vi "点位计算软件.vi"() -> ()   [LabVIEW 2020]
panel:
  in  "计算":bool
  out "error out":errorcluster
  in  "保存路径":path=path "D:/上下限/输入输出.ini" caption="配置文件的路径"
  in  "保存":bool
  in  "退出":bool
  in  "Tab Control":T1(tab)
  in  "Y 13":dbl
  in  "X 13":dbl
  in  "Y 12":dbl
  in  "X 12":dbl
  in  "Y 11":dbl
  in  "X 11":dbl
  in  "Y 10":dbl
  in  "X 10":dbl
  in  "Y 9":dbl
  in  "X 9":dbl
  in  "Y 8":dbl
  in  "X 8":dbl
  in  "Y 7":dbl
  in  "X 7":dbl
  in  "Y 6":dbl
  in  "X 6":dbl
  in  "Y 4":dbl
  in  "X 4":dbl
  in  "Y 5":dbl
  in  "X 5":dbl
  in  "Y 3":dbl
  in  "X 3":dbl
  in  "X 2":dbl
  in  "Y 2":dbl
  in  "Y 1":dbl
  in  "X 1":dbl
  in  "Y0":dbl
  in  "X 0":dbl
  out "?":bool
  out "?":bool
  out "?":bool
  out "?":bool
  out "?":bool
  out "?":bool
  out "?":bool
  out "?":bool
  out "?":bool
  out "?":bool
  out "?":bool
  out "?":bool
  out "?":bool
  out "?":bool
  in  "右侧边缘X坐标":dbl=2000.0 format="%#.3f"
  in  "左侧边缘X坐标":dbl=1000.0
  in  "上侧边缘Y坐标":dbl=1000.0
  in  "下侧边缘Y坐标":dbl=2000.0
  in  "产品宽度":dbl=23.67 format="%#_13g"
  in  "产品长度":dbl=13.3 format="%#_13g"
  in  "左侧边缘X坐标":dbl=1000.0
  in  "右侧边缘X坐标":dbl=2000.0 format="%#.3f"
  in  "上侧边缘Y坐标":dbl=1000.0
  in  "下侧边缘Y坐标":dbl=2000.0
  in  "X 8":dbl
  in  "Y 8":dbl
  in  "X 7":dbl
  in  "Y 7":dbl
  in  "X 6":dbl
  in  "Y 6":dbl
  in  "X 5":dbl
  in  "Y 5":dbl
  in  "X 4":dbl
  in  "Y 4":dbl
  in  "X 3":dbl
  in  "Y 3":dbl
  in  "Y 2":dbl
  in  "X 2":dbl
  in  "X 1":dbl
  in  "Y 1":dbl
  in  "X 0":dbl
  in  "Y 0":dbl
  out "?":bool
  out "?":bool
  out "?":bool
  out "?":bool
  out "?":bool
  out "?":bool
  out "?":bool
  out "?":bool
  out "?":bool
  out "?":bool
  out "?":bool
  out "?":bool
  out "?":bool
  out "?":bool
  out "?":bool
  out "?":bool
  out "?":bool
  out "?":bool
  out "?":bool
  out "?":bool
  out "?":bool
  out "?":bool
  out "?":bool
  out "X 0":dbl format="%#.3f"
  out "Y 0":dbl format="%#.3f"
  out "X 1":dbl format="%#.3f"
  out "Y 1":dbl format="%#.3f"
  out "Y 2":dbl format="%#.3f"
  out "X 2":dbl format="%#.3f"
  out "X 3":dbl format="%#.3f"
  out "Y 3":dbl format="%#.3f"
  out "X 5":dbl format="%#.3f"
  out "Y 5":dbl format="%#.3f"
  out "X 4":dbl format="%#.3f"
  out "Y 4":dbl format="%#.3f"
  out "X 6":dbl format="%#.3f"
  out "Y 6":dbl format="%#.3f"
  out "X 7":dbl format="%#.3f"
  out "Y 7":dbl format="%#.3f"
  out "X 8":dbl format="%#.3f"
  out "Y 8":dbl format="%#.3f"
  out "X 9":dbl format="%#.3f"
  out "Y 9":dbl format="%#.3f"
  out "X 10":dbl format="%#.3f"
  out "Y 10":dbl format="%#.3f"
  out "X 11":dbl format="%#.3f"
  out "Y 11":dbl format="%#.3f"
  out "X 12":dbl format="%#.3f"
  out "Y 12":dbl format="%#.3f"
  out "X 13":dbl format="%#.3f"
  out "Y 13":dbl format="%#.3f"
  out "?":bool
  out "?":bool
  out "?":bool
  out "?":bool
  out "?":bool
  out "?":bool
  out "?":bool
  out "?":bool
  out "?":bool
  out "Y 0":dbl format="%#.3f"
  out "X 0":dbl format="%#.3f"
  out "Y 1":dbl format="%#.3f"
  out "X 1":dbl format="%#.3f"
  out "X 2":dbl format="%#.3f"
  out "Y 2":dbl format="%#.3f"
  out "Y 3":dbl format="%#.3f"
  out "X 3":dbl format="%#.3f"
  out "Y 4":dbl format="%#.3f"
  out "X 4":dbl format="%#.3f"
  out "Y 5":dbl format="%#.3f"
  out "X 5":dbl format="%#.3f"
  out "Y 6":dbl format="%#.3f"
  out "X 6":dbl format="%#.3f"
  out "Y 7":dbl format="%#.3f"
  out "X 7":dbl format="%#.3f"
  out "Y 8":dbl format="%#.3f"
  out "X 8":dbl format="%#.3f"
  out "Y 13":dbl format="%#.3f"
  out "X 13":dbl format="%#.3f"
  out "Y 12":dbl format="%#.3f"
  out "X 12":dbl format="%#.3f"
  out "Y 11":dbl format="%#.3f"
  out "X 11":dbl format="%#.3f"
  out "Y 10":dbl format="%#.3f"
  out "X 10":dbl format="%#.3f"
  out "Y 9":dbl format="%#.3f"
  out "X 9":dbl format="%#.3f"
  out "Y 8":dbl format="%#.3f"
  out "X 8":dbl format="%#.3f"
  out "Y 7":dbl format="%#.3f"
  out "X 7":dbl format="%#.3f"
  out "Y 6":dbl format="%#.3f"
  out "X 6":dbl format="%#.3f"
  out "Y 4":dbl format="%#.3f"
  out "X 4":dbl format="%#.3f"
  out "Y 5":dbl format="%#.3f"
  out "X 5":dbl format="%#.3f"
  out "Y 3":dbl format="%#.3f"
  out "X 3":dbl format="%#.3f"
  out "X 2":dbl format="%#.3f"
  out "Y 2":dbl format="%#.3f"
  out "Y 1":dbl format="%#.3f"
  out "X 1":dbl format="%#.3f"
  out "Y 0":dbl format="%#.3f"
  out "X 0":dbl format="%#.3f"
  out "?":bool
  out "?":bool
  out "?":bool
  out "?":bool
  out "?":bool
  out "?":bool
  out "?":bool
  out "?":bool
  out "?":bool
  out "?":bool
  out "?":bool
  out "?":bool
  out "?":bool
  out "?":bool
  out "X 8":dbl format="%#.3f"
  out "Y 8":dbl format="%#.3f"
  out "X 7":dbl format="%#.3f"
  out "Y 7":dbl format="%#.3f"
  out "X 6":dbl format="%#.3f"
  out "Y 6":dbl format="%#.3f"
  out "X 5":dbl format="%#.3f"
  out "Y 5":dbl format="%#.3f"
  out "X 4":dbl format="%#.3f"
  out "Y 4":dbl format="%#.3f"
  out "X 3":dbl format="%#.3f"
  out "Y 3":dbl format="%#.3f"
  out "Y 2":dbl format="%#.3f"
  out "X 2":dbl format="%#.3f"
  out "X 1":dbl format="%#.3f"
  out "Y 1":dbl format="%#.3f"
  out "X 0":dbl format="%#.3f"
  out "Y 0":dbl format="%#.3f"
  out "?":bool
  out "?":bool
  out "?":bool
  out "?":bool
  out "?":bool
  out "?":bool
  out "?":bool
  out "?":bool
  out "?":bool
  # "产品1"
  # "产品2"
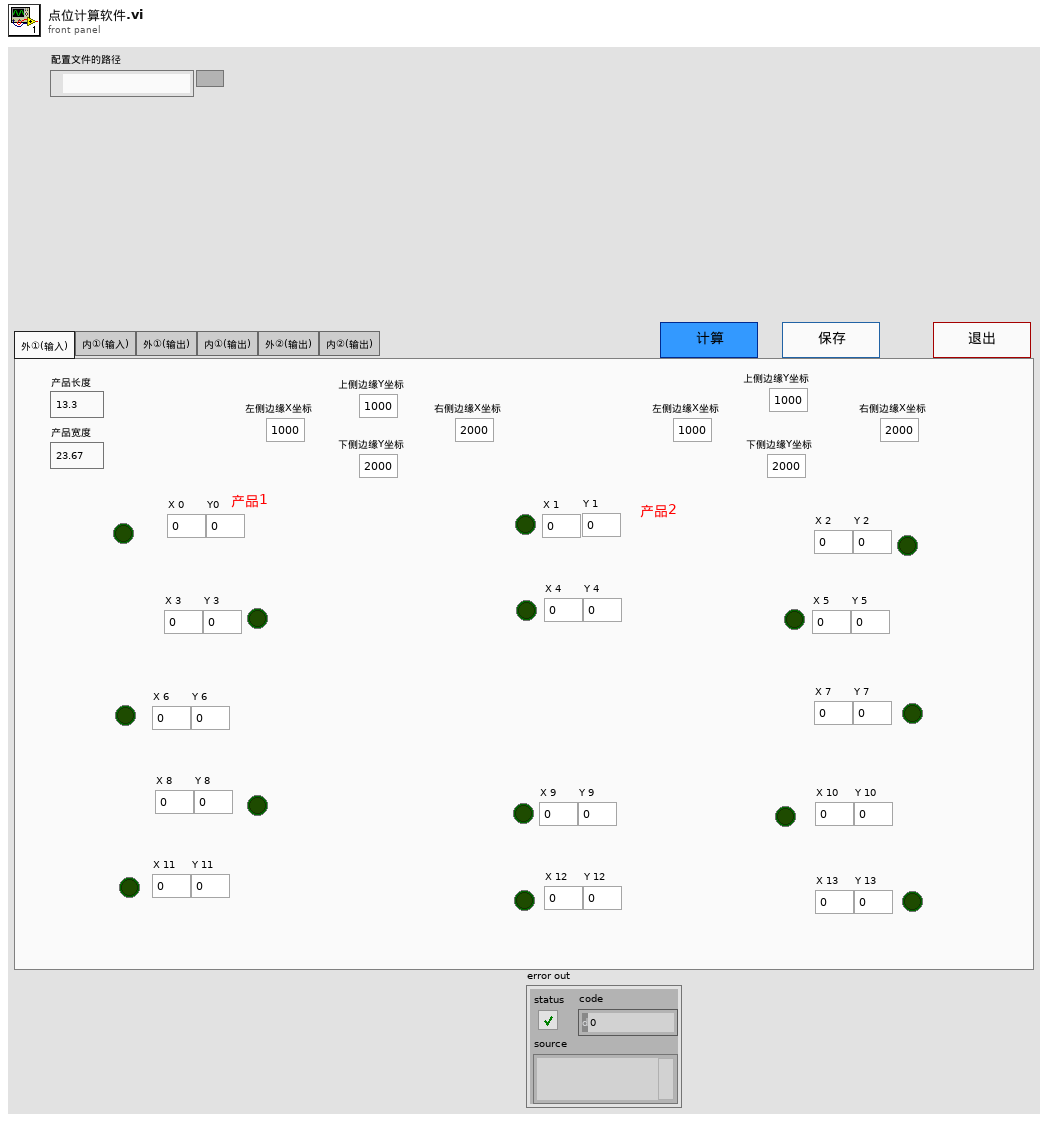
[diagram p1: front panel]
types:
  T1 = enum32{"外①(输入)", "内①(输入)", "外①(输出)", "内①(输出)", "外②(输出)", "内②(输出)"}
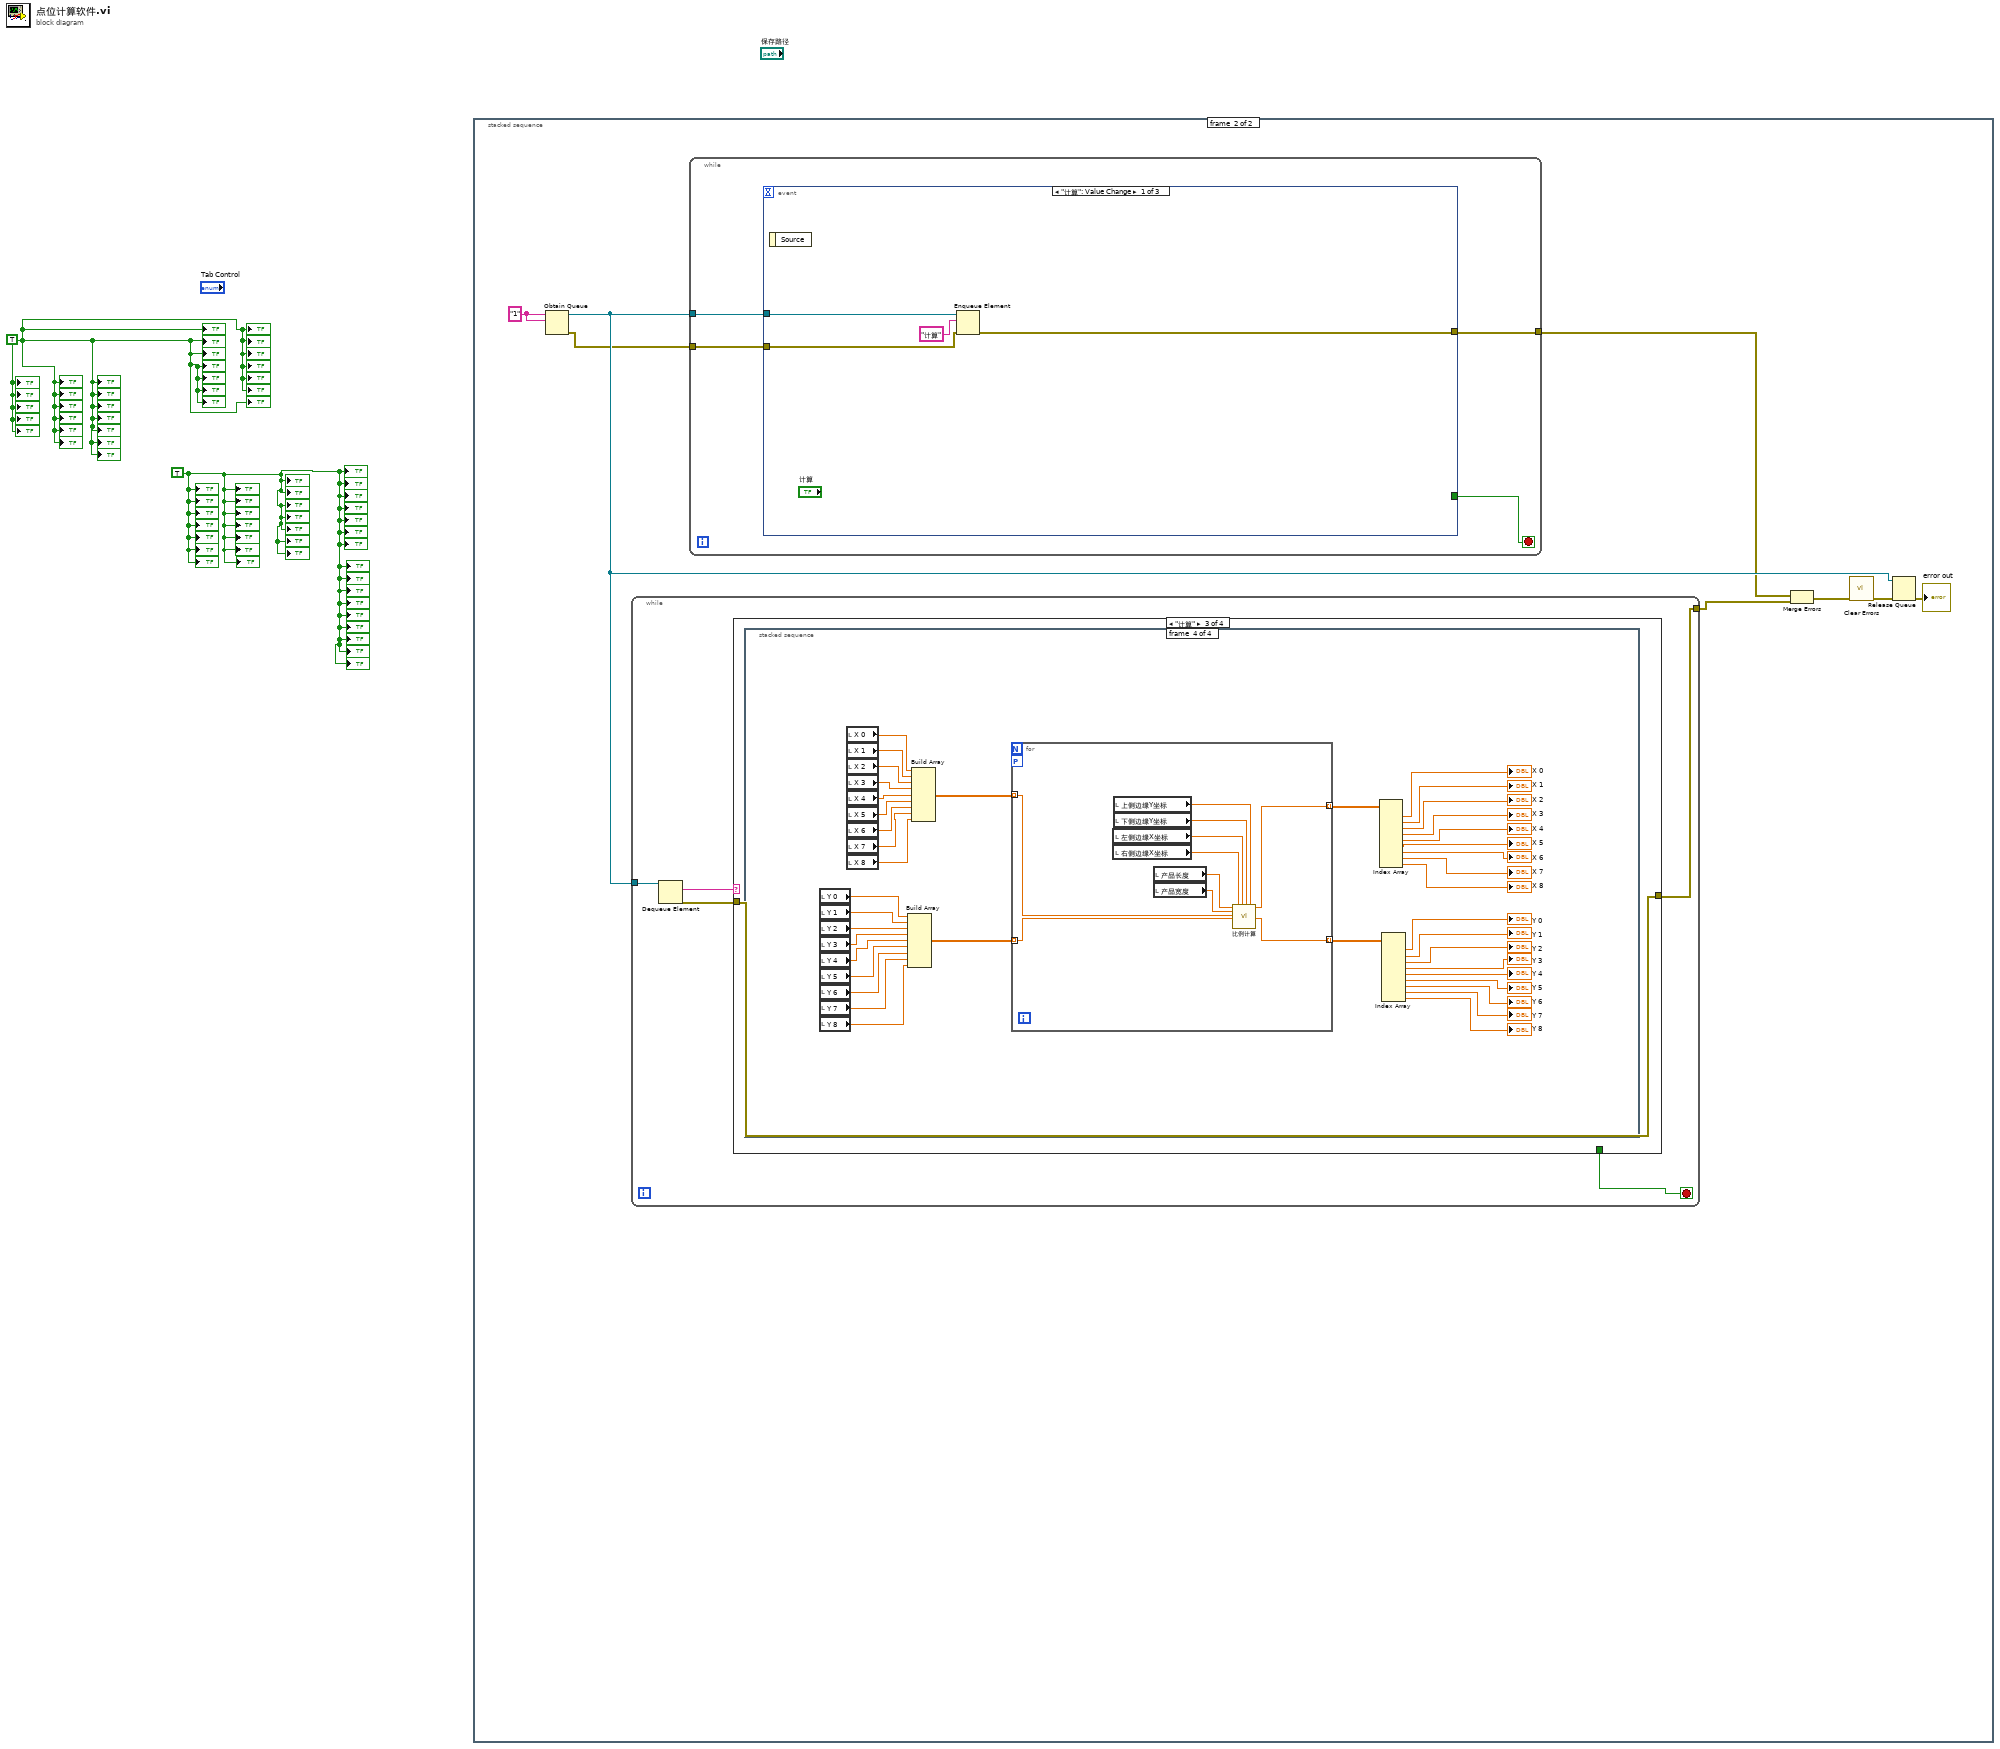
[diagram p0: block diagram]
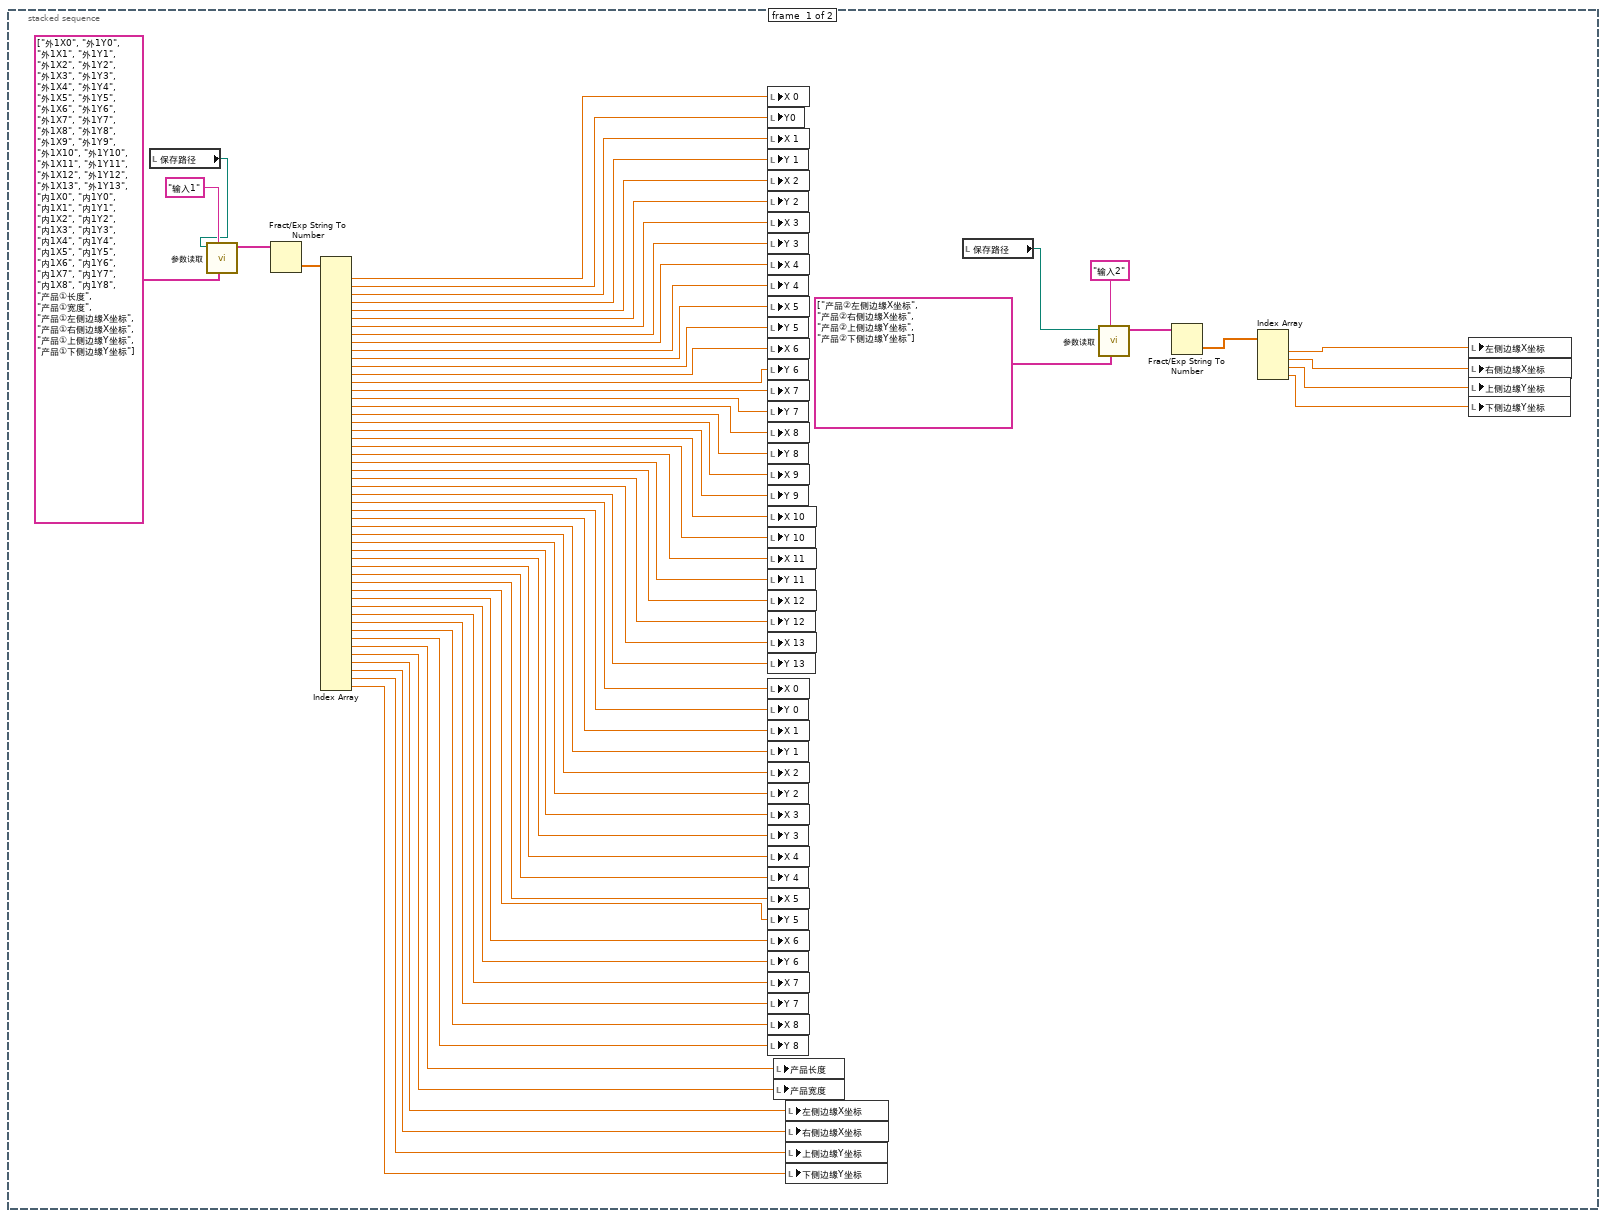
[diagram p2: hidden frame]
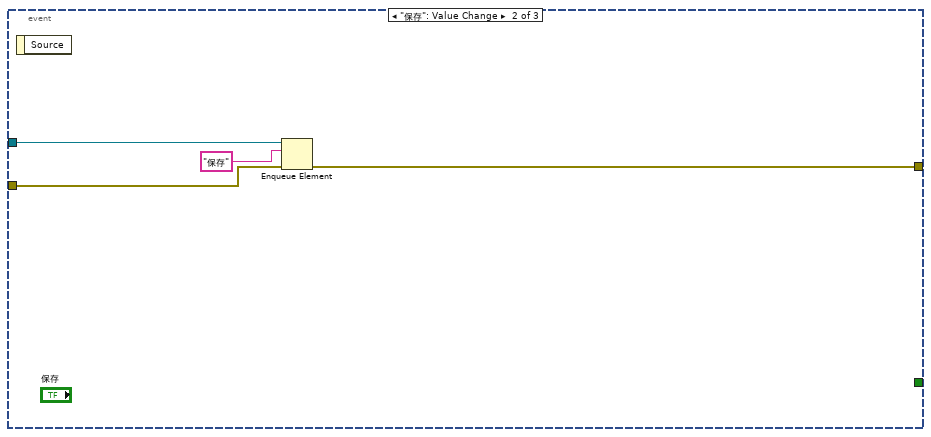
[diagram p3: hidden frame]
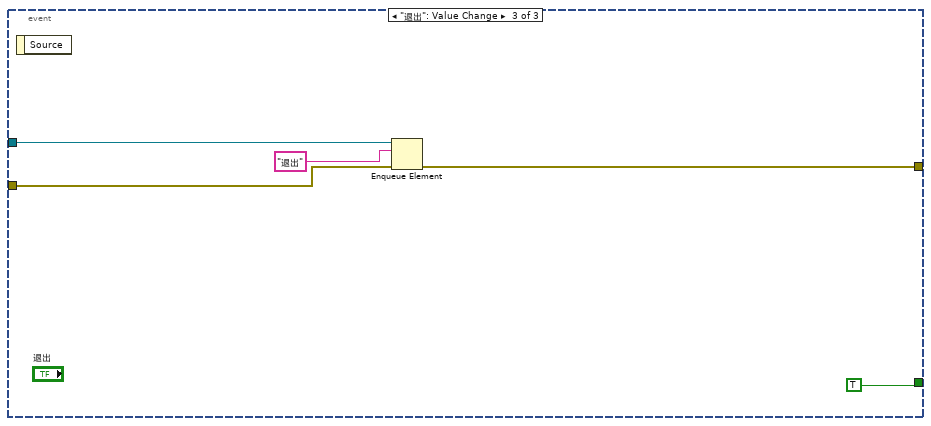
[diagram p4: hidden frame]
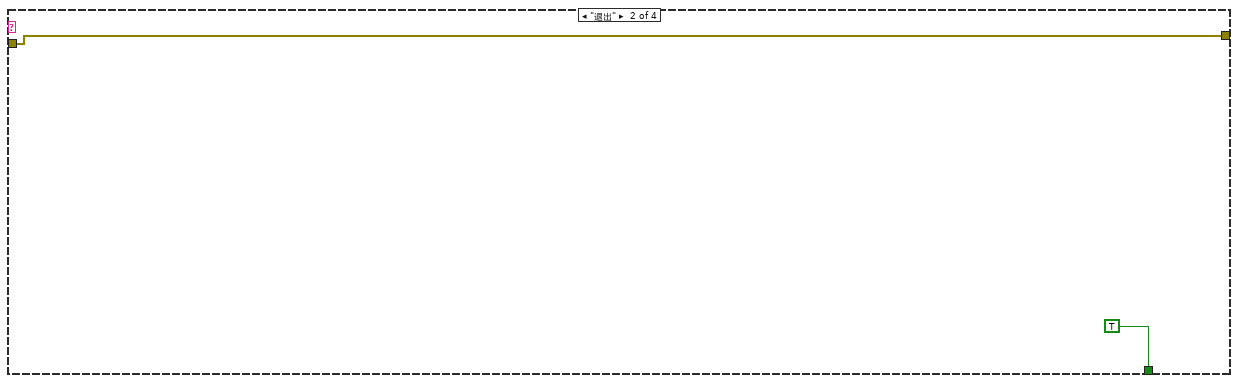
[diagram p6: hidden frame]
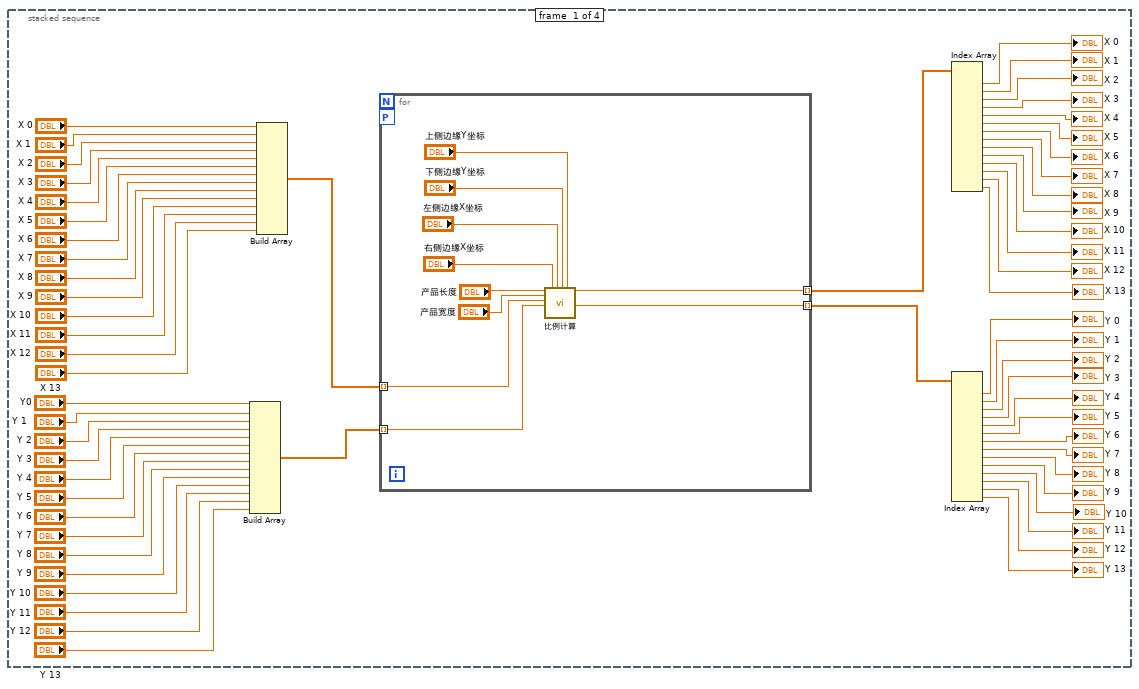
[diagram p7: hidden frame]
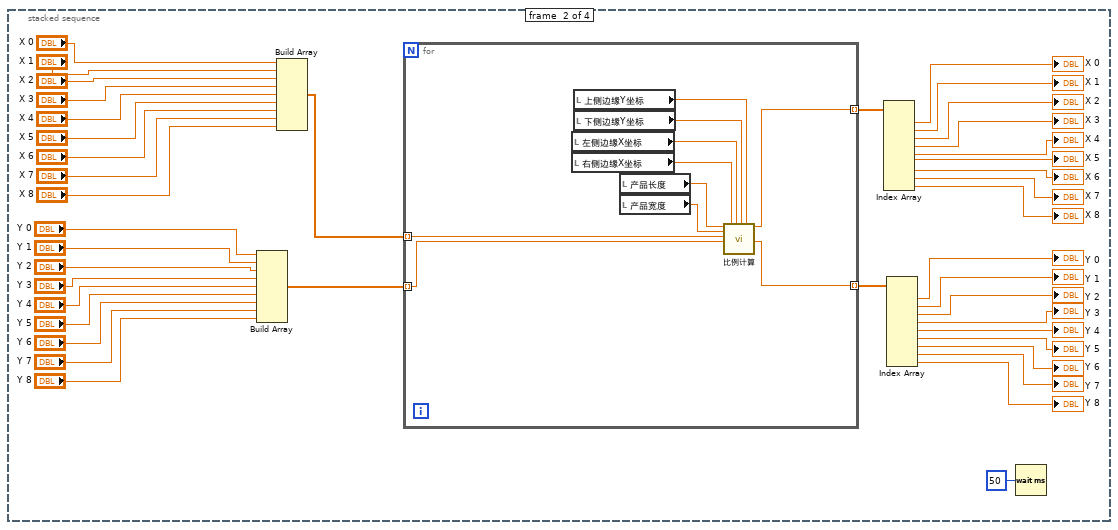
[diagram p8: hidden frame]
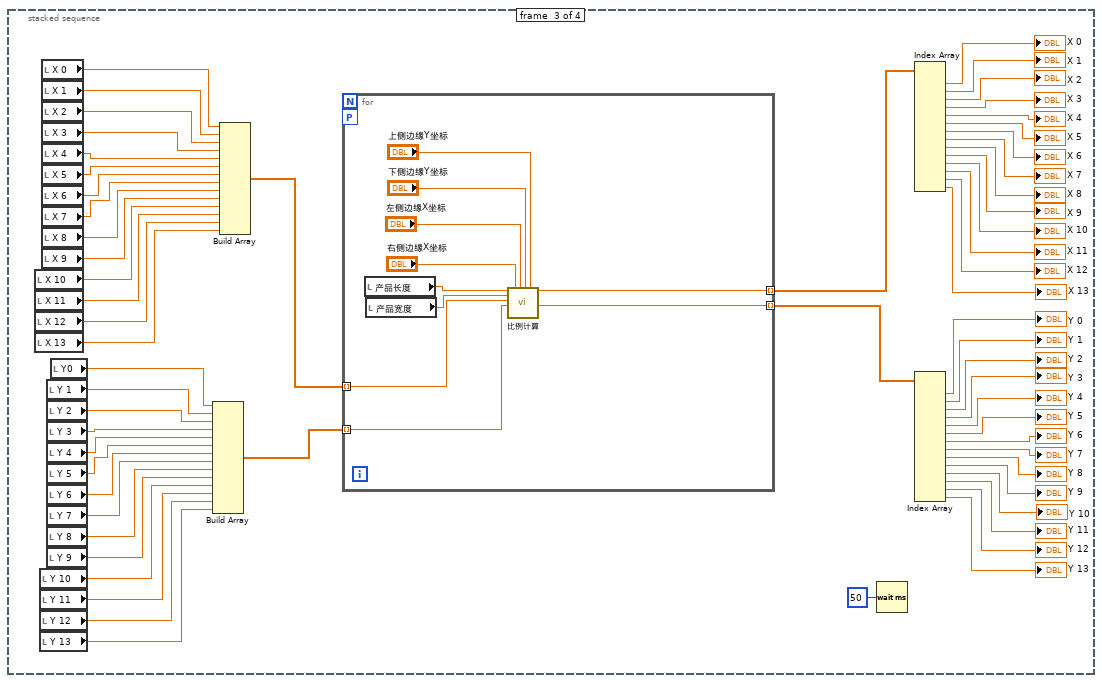
[diagram p9: hidden frame]
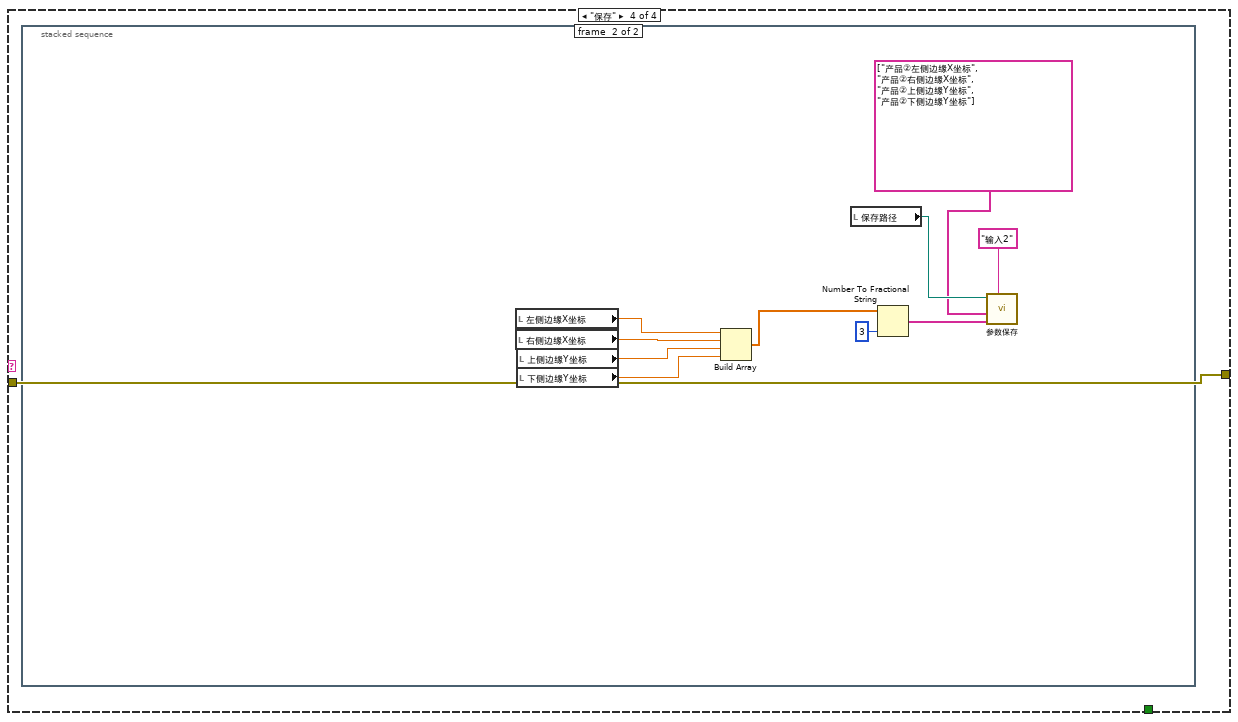
[diagram p10: hidden frame]
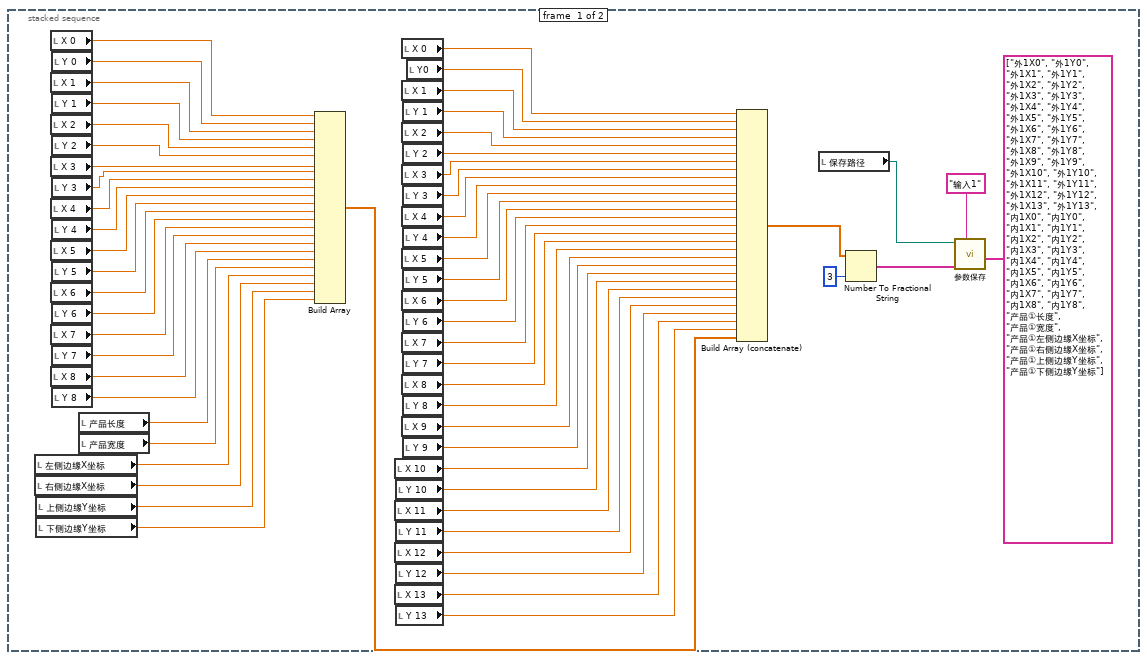
[diagram p11: hidden frame]
diagram:
  w1 = TRUE
  w2 = TRUE
  n1 = stacked-sequence {
    frame #0 {
      n2 = local read "保存路径"() -> (w19:path)
      n3 = call "参数读取.vi"("key names"=string[] ["外1X0", "外1Y0", "外1X1", "外1Y1", "外1X2", "外1Y2", "外1X3", "外1Y3", "外1X4", "外1Y4", "外1X5", "外1Y5", "外1X6", "外1Y6", "外1X7", "外1Y7", "外1X8", "外1Y8", "外1X9", "外1Y9", "外1X10", "外1Y10", "外1X11", "外1Y11", "外1X12", "外1Y12", "外1X13", "外1Y13", "内1X0", "内1Y0", "内1X1", "内1Y1", "内1X2", "内1Y2", "内1X3", "内1Y3", "内1X4", "内1Y4", "内1X5", "内1Y5", "内1X6", "内1Y6", "内1X7", "内1Y7", "内1X8", "内1Y8", "产品①长度", "产品①宽度", "产品①左侧边缘X坐标", "产品①右侧边缘X坐标", "产品①上侧边缘Y坐标", "产品①下侧边缘Y坐标"] ("键"), "段名"="输入1", "configuration file path"=w19) -> ("值"=w21:string[])  [unwired: 7 in, 1 out]
      n4 = Fract/Exp String To Number(string=w21) -> (number=w22:dbl[])  [unwired: 3 in, 1 out]
      n5 = Index Array(array=w22) -> (element #1=w23:dbl, element #2=w24:dbl, element #3=w25:dbl, element #4=w26:dbl, element #5=w27:dbl, element #6=w28:dbl, element #7=w29:dbl, element #8=w30:dbl, element #9=w31:dbl, element #10=w32:dbl, element #11=w33:dbl, element #12=w34:dbl, element #13=w35:dbl, element #14=w36:dbl, element #15=w37:dbl, element #16=w38:dbl, element #17=w39:dbl, element #18=w40:dbl, element #19=w41:dbl, element #20=w42:dbl, element #21=w43:dbl, element #22=w44:dbl, element #23=w45:dbl, element #24=w46:dbl, element #25=w47:dbl, element #26=w48:dbl, element #27=w49:dbl, element #28=w50:dbl, element #29=w51:dbl, element #30=w52:dbl, element #31=w53:dbl, element #32=w54:dbl, element #33=w55:dbl, element #34=w56:dbl, element #35=w57:dbl, element #36=w58:dbl, element #37=w59:dbl, element #38=w60:dbl, element #39=w61:dbl, element #40=w62:dbl, element #41=w63:dbl, element #42=w64:dbl, element #43=w65:dbl, element #44=w66:dbl, element #45=w67:dbl, element #46=w68:dbl, element #47=w17:dbl, element #48=w16:dbl, element #49=w15:dbl, element #50=w14:dbl, element #51=w13:dbl, element #52=w12:dbl)  [unwired: 52 in]
      n6 = local write "X 0"(w23) -> ()
      n7 = local write "Y0"(w24) -> ()
      n8 = local write "X 1"(w25) -> ()
      n9 = local write "Y 1"(w26) -> ()
      n10 = local write "X 2"(w27) -> ()
      n11 = local write "Y 2"(w28) -> ()
      n12 = local write "X 3"(w29) -> ()
      n13 = local write "Y 3"(w30) -> ()
      n14 = local write "X 4"(w31) -> ()
      n15 = local write "Y 4"(w32) -> ()
      n16 = local write "X 5"(w33) -> ()
      n17 = local write "Y 5"(w34) -> ()
      n18 = local write "X 6"(w35) -> ()
      n19 = local write "Y 6"(w36) -> ()
      n20 = local write "X 7"(w37) -> ()
      n21 = local write "Y 7"(w38) -> ()
      n22 = local write "X 8"(w39) -> ()
      n23 = local write "Y 8"(w40) -> ()
      n24 = local write "X 9"(w41) -> ()
      n25 = local write "Y 9"(w42) -> ()
      n26 = local write "X 10"(w43) -> ()
      n27 = local write "Y 10"(w44) -> ()
      n28 = local write "X 11"(w45) -> ()
      n29 = local write "Y 11"(w46) -> ()
      n30 = local write "X 12"(w47) -> ()
      n31 = local write "Y 12"(w48) -> ()
      n32 = local write "X 13"(w49) -> ()
      n33 = local write "Y 13"(w50) -> ()
      n34 = local write "X 0"(w51) -> ()
      n35 = local write "Y 0"(w52) -> ()
      n36 = local write "X 1"(w53) -> ()
      n37 = local write "Y 1"(w54) -> ()
      n38 = local write "X 2"(w55) -> ()
      n39 = local write "Y 2"(w56) -> ()
      n40 = local write "X 3"(w57) -> ()
      n41 = local write "Y 3"(w58) -> ()
      n42 = local write "X 4"(w59) -> ()
      n43 = local write "Y 4"(w60) -> ()
      n44 = local write "X 5"(w61) -> ()
      n45 = local write "Y 5"(w62) -> ()
      n46 = local write "X 6"(w63) -> ()
      n47 = local write "Y 6"(w64) -> ()
      n48 = local write "X 7"(w65) -> ()
      n49 = local write "Y 7"(w66) -> ()
      n50 = local write "X 8"(w67) -> ()
      n51 = local write "Y 8"(w68) -> ()
      n52 = local write "产品长度"(w17) -> ()
      n53 = local write "产品宽度"(w16) -> ()
      n54 = local write "左侧边缘X坐标"(w15) -> ()
      n55 = local write "右侧边缘X坐标"(w14) -> ()
      n56 = local write "上侧边缘Y坐标"(w13) -> ()
      n57 = local write "下侧边缘Y坐标"(w12) -> ()
      n58 = local read "保存路径"() -> (w11:path)
      n59 = call "参数读取.vi"("key names"=string[] ["产品②左侧边缘X坐标", "产品②右侧边缘X坐标", "产品②上侧边缘Y坐标", "产品②下侧边缘Y坐标"], "段名"="输入2", "configuration file path"=w11) -> ("值"=w9:string[])  [unwired: 7 in, 1 out]
      n60 = Fract/Exp String To Number(string=w9) -> (number=w4:dbl[])  [unwired: 3 in, 1 out]
      n61 = Index Array(array=w4) -> (element #1=w8:dbl, element #2=w7:dbl, element #3=w6:dbl, element #4=w5:dbl)  [unwired: 4 in]
      n62 = local write "左侧边缘X坐标"(w8) -> ()
      n63 = local write "右侧边缘X坐标"(w7) -> ()
      n64 = local write "上侧边缘Y坐标"(w6) -> ()
      n65 = local write "下侧边缘Y坐标"(w5) -> ()
    }
    frame #1 {
      w76 = "1" ("name (unnamed)")
      n66 = Obtain Queue(name (unnamed)=w76, element data type=w76) -> (queue out=w72:refnum<queue>, error out=w71:errorcluster)  [unwired: 3 in, 1 out]
      n67 = while {
        tunnel: w72 -> [w97]
        tunnel: [w95] -> w74
        stop <- w98 stop-if-true
        n68 = Dequeue Element(queue=w97) -> (element=w96:string, error out=w94:errorcluster)  [unwired: 2 in, 2 out]
        n69 = case shown="\"计算\"" w96 {
          tunnel: [_ TRUE _ _] -> w98
          tunnel: [w99 w100 w102 w345] -> w95
          tunnel: w94 -> [w99 w100 w102 w345]
          frame Default {
          }
          frame "退出" {
          }
          frame "计算" {
            n70 = stacked-sequence {
              frame #0 {
                n71 = Build Array("Y0", "Y 1", "Y 2", "Y 3", "Y 4", "Y 5", "Y 6", "Y 7", "Y 8", "Y 9", "Y 10", "Y 11", "Y 12", "Y 13") -> (w133:dbl[])
                n72 = Build Array("X 0", "X 1", "X 2", "X 3", "X 4", "X 5", "X 6", "X 7", "X 8", "X 9", "X 10", "X 11", "X 12", "X 13") -> (w148:dbl[])
                n73 = for {
                  workers-P: _ -> [_]
                  tunnel: w148 -> [w166] mode=indexing
                  tunnel: w133 -> [w165] mode=indexing
                  tunnel: [w164] -> w132 mode=indexing
                  tunnel: [w163] -> w119 mode=indexing
                  n74 = call "比例计算.vi"("产品长度"="产品长度", "产品宽度"="产品宽度", "真实X"=w166, "真实Y"=w165, "产品1右侧边缘X坐标"="右侧边缘X坐标", "产品1左侧边缘X坐标"="左侧边缘X坐标", "产品1下侧边缘Y坐标"="下侧边缘Y坐标", "产品1上侧边缘Y坐标"="上侧边缘Y坐标") -> ("X"=w164:dbl, "Y"=w163:dbl)  [unwired: 10 in]
                }
                n75 = Index Array(array=w132) -> (element #1=→"X 0":dbl, element #2=→"X 1":dbl, element #3=→"X 2":dbl, element #4=→"X 3":dbl, element #5=→"X 4":dbl, element #6=→"X 5":dbl, element #7=→"X 6":dbl, element #8=→"X 7":dbl, element #9=→"X 8":dbl, element #10=→"X 9":dbl, element #11=→"X 10":dbl, element #12=→"X 11":dbl, element #13=→"X 12":dbl, element #14=→"X 13":dbl)  [unwired: 14 in]
                n76 = Index Array(array=w119) -> (element #1=→"Y 0":dbl, element #2=→"Y 1":dbl, element #3=→"Y 2":dbl, element #4=→"Y 3":dbl, element #5=→"Y 4":dbl, element #6=→"Y 5":dbl, element #7=→"Y 6":dbl, element #8=→"Y 7":dbl, element #9=→"Y 8":dbl, element #10=→"Y 9":dbl, element #11=→"Y 10":dbl, element #12=→"Y 11":dbl, element #13=→"Y 12":dbl, element #14=→"Y 13":dbl)  [unwired: 14 in]
              }
              frame #1 {
                n77 = Build Array("Y 0", "Y 1", "Y 2", "Y 3", "Y 4", "Y 5", "Y 6", "Y 7", "Y 8") -> (w193:dbl[])
                n78 = Build Array("X 0", "X 1", "X 2", "X 3", "X 4", "X 5", "X 6", "X 7", "X 8") -> (w192:dbl[])
                n79 = for {
                  tunnel: w192 -> [w217] mode=indexing
                  tunnel: w193 -> [w216] mode=indexing
                  tunnel: [w215] -> w194 mode=indexing
                  tunnel: [w214] -> w204 mode=indexing
                  n80 = local read "左侧边缘X坐标"() -> (w221:dbl)
                  n81 = local read "右侧边缘X坐标"() -> (w220:dbl)
                  n82 = local read "上侧边缘Y坐标"() -> (w223:dbl)
                  n83 = local read "下侧边缘Y坐标"() -> (w222:dbl)
                  n84 = local read "产品长度"() -> (w219:dbl)
                  n85 = local read "产品宽度"() -> (w218:dbl)
                  n86 = call "比例计算.vi"("产品长度"=w219, "产品宽度"=w218, "真实X"=w217, "真实Y"=w216, "产品1右侧边缘X坐标"=w220, "产品1左侧边缘X坐标"=w221, "产品1下侧边缘Y坐标"=w222, "产品1上侧边缘Y坐标"=w223) -> ("X"=w215:dbl, "Y"=w214:dbl)  [unwired: 10 in]
                }
                n87 = Index Array(array=w194) -> (element #1=→"X 0":dbl, element #2=→"X 1":dbl, element #3=→"X 2":dbl, element #4=→"X 3":dbl, element #5=→"X 4":dbl, element #6=→"X 5":dbl, element #7=→"X 6":dbl, element #8=→"X 7":dbl, element #9=→"X 8":dbl)  [unwired: 9 in]
                n88 = Index Array(array=w204) -> (element #1=→"Y 0":dbl, element #2=→"Y 1":dbl, element #3=→"Y 2":dbl, element #4=→"Y 3":dbl, element #5=→"Y 4":dbl, element #6=→"Y 5":dbl, element #7=→"Y 6":dbl, element #8=→"Y 7":dbl, element #9=→"Y 8":dbl)  [unwired: 9 in]
                n89 = Wait (ms)(milliseconds to wait=u32 50) -> ()  [unwired: 1 out]
              }
              frame #2 {
                n90 = local read "X 10"() -> (w242:dbl)
                n91 = local read "X 11"() -> (w241:dbl)
                n92 = local read "X 12"() -> (w240:dbl)
                n93 = local read "X 13"() -> (w239:dbl)
                n94 = local read "Y 10"() -> (w228:dbl)
                n95 = local read "Y 11"() -> (w227:dbl)
                n96 = local read "Y 12"() -> (w226:dbl)
                n97 = local read "Y 13"() -> (w225:dbl)
                n98 = local read "X 0"() -> (w252:dbl)
                n99 = local read "X 1"() -> (w251:dbl)
                n100 = local read "X 2"() -> (w250:dbl)
                n101 = local read "X 3"() -> (w249:dbl)
                n102 = local read "X 4"() -> (w248:dbl)
                n103 = local read "X 5"() -> (w247:dbl)
                n104 = local read "X 6"() -> (w246:dbl)
                n105 = local read "X 7"() -> (w245:dbl)
                n106 = local read "X 8"() -> (w244:dbl)
                n107 = local read "X 9"() -> (w243:dbl)
                n108 = local read "Y 1"() -> (w237:dbl)
                n109 = local read "Y 2"() -> (w236:dbl)
                n110 = local read "Y 3"() -> (w235:dbl)
                n111 = local read "Y 4"() -> (w234:dbl)
                n112 = local read "Y 5"() -> (w233:dbl)
                n113 = local read "Y 6"() -> (w232:dbl)
                n114 = local read "Y 7"() -> (w231:dbl)
                n115 = local read "Y 8"() -> (w230:dbl)
                n116 = local read "Y 9"() -> (w229:dbl)
                n117 = local read "Y0"() -> (w238:dbl)
                n118 = Build Array(w238, w237, w236, w235, w234, w233, w232, w231, w230, w229, w228, w227, w226, w225) -> (w283:dbl[])
                n119 = Build Array(w252, w251, w250, w249, w248, w247, w246, w245, w244, w243, w242, w241, w240, w239) -> (w284:dbl[])
                n120 = for {
                  workers-P: _ -> [_]
                  tunnel: w284 -> [w286] mode=indexing
                  tunnel: w283 -> [w285] mode=indexing
                  tunnel: [w290] -> w282 mode=indexing
                  tunnel: [w289] -> w269 mode=indexing
                  n121 = local read "产品长度"() -> (w288:dbl)
                  n122 = local read "产品宽度"() -> (w287:dbl)
                  n123 = call "比例计算.vi"("产品长度"=w288, "产品宽度"=w287, "真实X"=w286, "真实Y"=w285, "产品1右侧边缘X坐标"="右侧边缘X坐标", "产品1左侧边缘X坐标"="左侧边缘X坐标", "产品1下侧边缘Y坐标"="下侧边缘Y坐标", "产品1上侧边缘Y坐标"="上侧边缘Y坐标") -> ("X"=w290:dbl, "Y"=w289:dbl)  [unwired: 10 in]
                }
                n124 = Wait (ms)(milliseconds to wait=u32 50) -> ()  [unwired: 1 out]
                n125 = Index Array(array=w282) -> (element #1=→"X 0":dbl, element #2=→"X 1":dbl, element #3=→"X 2":dbl, element #4=→"X 3":dbl, element #5=→"X 4":dbl, element #6=→"X 5":dbl, element #7=→"X 6":dbl, element #8=→"X 7":dbl, element #9=→"X 8":dbl, element #10=→"X 9":dbl, element #11=→"X 10":dbl, element #12=→"X 11":dbl, element #13=→"X 12":dbl, element #14=→"X 13":dbl)  [unwired: 14 in]
                n126 = Index Array(array=w269) -> (element #1=→"Y 0":dbl, element #2=→"Y 1":dbl, element #3=→"Y 2":dbl, element #4=→"Y 3":dbl, element #5=→"Y 4":dbl, element #6=→"Y 5":dbl, element #7=→"Y 6":dbl, element #8=→"Y 7":dbl, element #9=→"Y 8":dbl, element #10=→"Y 9":dbl, element #11=→"Y 10":dbl, element #12=→"Y 11":dbl, element #13=→"Y 12":dbl, element #14=→"Y 13":dbl)  [unwired: 14 in]
              }
              frame #3 {
                n127 = local read "Y 0"() -> (w303:dbl)
                n128 = local read "Y 1"() -> (w302:dbl)
                n129 = local read "Y 2"() -> (w301:dbl)
                n130 = local read "Y 3"() -> (w300:dbl)
                n131 = local read "Y 4"() -> (w299:dbl)
                n132 = local read "Y 5"() -> (w298:dbl)
                n133 = local read "Y 6"() -> (w297:dbl)
                n134 = local read "Y 7"() -> (w296:dbl)
                n135 = local read "Y 8"() -> (w295:dbl)
                n136 = local read "X 0"() -> (w312:dbl)
                n137 = local read "X 1"() -> (w311:dbl)
                n138 = local read "X 2"() -> (w310:dbl)
                n139 = local read "X 3"() -> (w309:dbl)
                n140 = local read "X 4"() -> (w308:dbl)
                n141 = local read "X 5"() -> (w307:dbl)
                n142 = local read "X 6"() -> (w306:dbl)
                n143 = local read "X 7"() -> (w305:dbl)
                n144 = local read "X 8"() -> (w304:dbl)
                n145 = Build Array(w303, w302, w301, w300, w299, w298, w297, w296, w295) -> (w314:dbl[])
                n146 = Build Array(w312, w311, w310, w309, w308, w307, w306, w305, w304) -> (w313:dbl[])
                n147 = for {
                  workers-P: _ -> [_]
                  tunnel: w313 -> [w340] mode=indexing
                  tunnel: w314 -> [w339] mode=indexing
                  tunnel: [w342] -> w315 mode=indexing
                  tunnel: [w341] -> w316 mode=indexing
                  n148 = local read "左侧边缘X坐标"() -> (w336:dbl)
                  n149 = local read "右侧边缘X坐标"() -> (w335:dbl)
                  n150 = local read "上侧边缘Y坐标"() -> (w338:dbl)
                  n151 = local read "下侧边缘Y坐标"() -> (w337:dbl)
                  n152 = local read "产品长度"() -> (w343:dbl)
                  n153 = local read "产品宽度"() -> (w344:dbl)
                  n154 = call "比例计算.vi"("产品长度"=w343, "产品宽度"=w344, "真实X"=w340, "真实Y"=w339, "产品1右侧边缘X坐标"=w335, "产品1左侧边缘X坐标"=w336, "产品1下侧边缘Y坐标"=w337, "产品1上侧边缘Y坐标"=w338) -> ("X"=w342:dbl, "Y"=w341:dbl)  [unwired: 10 in]
                }
                n155 = Index Array(array=w315) -> (element #1=→"X 0":dbl, element #2=→"X 1":dbl, element #3=→"X 2":dbl, element #4=→"X 3":dbl, element #5=→"X 4":dbl, element #6=→"X 5":dbl, element #7=→"X 6":dbl, element #8=→"X 7":dbl, element #9=→"X 8":dbl)  [unwired: 9 in]
                n156 = Index Array(array=w316) -> (element #1=→"Y 0":dbl, element #2=→"Y 1":dbl, element #3=→"Y 2":dbl, element #4=→"Y 3":dbl, element #5=→"Y 4":dbl, element #6=→"Y 5":dbl, element #7=→"Y 6":dbl, element #8=→"Y 7":dbl, element #9=→"Y 8":dbl)  [unwired: 9 in]
              }
            }
          }
          frame "保存" {
            n157 = stacked-sequence {
              frame #0 {
                n158 = local read "左侧边缘X坐标"() -> (w349:dbl)
                n159 = local read "右侧边缘X坐标"() -> (w348:dbl)
                n160 = local read "上侧边缘Y坐标"() -> (w347:dbl)
                n161 = local read "下侧边缘Y坐标"() -> (w346:dbl)
                n162 = local read "X 0"() -> (w374:dbl)
                n163 = local read "X 1"() -> (w372:dbl)
                n164 = local read "X 2"() -> (w370:dbl)
                n165 = local read "X 3"() -> (w368:dbl)
                n166 = local read "X 4"() -> (w366:dbl)
                n167 = local read "X 5"() -> (w364:dbl)
                n168 = local read "X 6"() -> (w362:dbl)
                n169 = local read "X 7"() -> (w360:dbl)
                n170 = local read "X 8"() -> (w358:dbl)
                n171 = local read "Y 0"() -> (w373:dbl)
                n172 = local read "Y 1"() -> (w371:dbl)
                n173 = local read "Y 2"() -> (w369:dbl)
                n174 = local read "Y 3"() -> (w367:dbl)
                n175 = local read "Y 4"() -> (w365:dbl)
                n176 = local read "Y 5"() -> (w363:dbl)
                n177 = local read "Y 6"() -> (w361:dbl)
                n178 = local read "Y 7"() -> (w359:dbl)
                n179 = local read "Y 8"() -> (w357:dbl)
                n180 = local read "产品长度"() -> (w351:dbl)
                n181 = local read "产品宽度"() -> (w350:dbl)
                n182 = Build Array(w374, w373, w372, w371, w370, w369, w368, w367, w366, w365, w364, w363, w362, w361, w360, w359, w358, w357, w351, w350, w349, w348, w347, w346) -> (w356:dbl[])
                n183 = local read "X 10"() -> (w382:dbl)
                n184 = local read "X 11"() -> (w380:dbl)
                n185 = local read "X 12"() -> (w378:dbl)
                n186 = local read "X 13"() -> (w376:dbl)
                n187 = local read "Y 10"() -> (w381:dbl)
                n188 = local read "Y 11"() -> (w379:dbl)
                n189 = local read "Y 12"() -> (w377:dbl)
                n190 = local read "Y 13"() -> (w375:dbl)
                n191 = local read "X 0"() -> (w402:dbl)
                n192 = local read "X 1"() -> (w400:dbl)
                n193 = local read "X 2"() -> (w398:dbl)
                n194 = local read "X 3"() -> (w396:dbl)
                n195 = local read "X 4"() -> (w394:dbl)
                n196 = local read "X 5"() -> (w392:dbl)
                n197 = local read "X 6"() -> (w390:dbl)
                n198 = local read "X 7"() -> (w388:dbl)
                n199 = local read "X 8"() -> (w386:dbl)
                n200 = local read "X 9"() -> (w384:dbl)
                n201 = local read "Y 1"() -> (w399:dbl)
                n202 = local read "Y 2"() -> (w397:dbl)
                n203 = local read "Y 3"() -> (w395:dbl)
                n204 = local read "Y 4"() -> (w393:dbl)
                n205 = local read "Y 5"() -> (w391:dbl)
                n206 = local read "Y 6"() -> (w389:dbl)
                n207 = local read "Y 7"() -> (w387:dbl)
                n208 = local read "Y 8"() -> (w385:dbl)
                n209 = local read "Y 9"() -> (w383:dbl)
                n210 = local read "Y0"() -> (w401:dbl)
                n211 = Build Array (concatenate)(w402, w401, w400, w399, w398, w397, w396, w395, w394, w393, w392, w391, w390, w389, w388, w387, w386, w385, w384, w383, w382, w381, w380, w379, w378, w377, w376, w375, w356) -> (w355:dbl[])
                n212 = local read "保存路径"() -> (w352:path)
                n213 = Number To Fractional String(number=w355, precision (6)=i16 3) -> (F-format string=w354:string[])  [unwired: 2 in]
                n214 = call "参数保存.vi"("段名"="输入1", "值"=w354, "键"=string[] ["外1X0", "外1Y0", "外1X1", "外1Y1", "外1X2", "外1Y2", "外1X3", "外1Y3", "外1X4", "外1Y4", "外1X5", "外1Y5", "外1X6", "外1Y6", "外1X7", "外1Y7", "外1X8", "外1Y8", "外1X9", "外1Y9", "外1X10", "外1Y10", "外1X11", "外1Y11", "外1X12", "外1Y12", "外1X13", "外1Y13", "内1X0", "内1Y0", "内1X1", "内1Y1", "内1X2", "内1Y2", "内1X3", "内1Y3", "内1X4", "内1Y4", "内1X5", "内1Y5", "内1X6", "内1Y6", "内1X7", "内1Y7", "内1X8", "内1Y8", "产品①长度", "产品①宽度", "产品①左侧边缘X坐标", "产品①右侧边缘X坐标", "产品①上侧边缘Y坐标", "产品①下侧边缘Y坐标"], "configuration file path"=w352) -> ()  [unwired: 8 in]
              }
              frame #1 {
                n215 = local read "左侧边缘X坐标"() -> (w411:dbl)
                n216 = local read "右侧边缘X坐标"() -> (w410:dbl)
                n217 = local read "上侧边缘Y坐标"() -> (w409:dbl)
                n218 = local read "下侧边缘Y坐标"() -> (w408:dbl)
                n219 = Build Array(w411, w410, w409, w408) -> (w406:dbl[])
                n220 = local read "保存路径"() -> (w414:path)
                n221 = Number To Fractional String(number=w406, precision (6)=i16 3) -> (F-format string=w405:string[])  [unwired: 2 in]
                n222 = call "参数保存.vi"("段名"="输入2", "值"=w405, "键"=string[] ["产品②左侧边缘X坐标", "产品②右侧边缘X坐标", "产品②上侧边缘Y坐标", "产品②下侧边缘Y坐标"], "configuration file path"=w414) -> ()  [unwired: 8 in]
              }
            }
          }
        }
      }
      n223 = while {
        tunnel: w72 -> [w80]
        tunnel: w71 -> [w78]
        tunnel: [w77] -> w70
        stop <- w79 stop-if-true
        n224 = event shown="[0] \"计算\": Value Change" {
          selector: _ -> [_ _ _]
          dyn-events: _ -> [_ _ _]
          timeout: _ -> [_ _ _]
          tunnel: w80 -> [w83 w87 w93]
          tunnel: [w82 w86 w92] -> w77
          tunnel: [_ _ TRUE] -> w79
          tunnel: w78 -> [w81 w85 w89]
          event "计算": Value Change {
            n225 = event-data() -> ()  [unwired: 1 in, 1 out]
            n226 = Enqueue Element(queue=w83, element="计算", error in (no error)=w81) -> (error out=w82:errorcluster)  [unwired: 1 in, 2 out]
          }
          event "保存": Value Change {
            n227 = event-data() -> ()  [unwired: 1 in, 1 out]
            n228 = Enqueue Element(queue=w87, element="保存", error in (no error)=w85) -> (error out=w86:errorcluster)  [unwired: 1 in, 2 out]
          }
          event "退出": Value Change {
            n229 = event-data() -> ()  [unwired: 1 in, 1 out]
            n230 = Enqueue Element(queue=w93, element="退出", error in (no error)=w89) -> (error out=w92:errorcluster)  [unwired: 1 in, 2 out]
          }
        }
      }
      n231 = Merge Errors(w70, w74) -> (w75:errorcluster)
      n232 = call <vilib>:"Clear Errors.vi"("error in (no error)"=w75) -> ("error out"=w73:errorcluster)  [unwired: 5 in, 1 out]
      n233 = Release Queue(queue=w72, error in (no error)=w73) -> (error out=→"error out":errorcluster)  [unwired: 1 in, 2 out]
    }
  }
  "?" <- w2
  "?" <- w2
  "?" <- w2
  "?" <- w2
  "?" <- w2
  "?" <- w2
  "?" <- w2
  "?" <- w2
  "?" <- w2
  "?" <- w2
  "?" <- w2
  "?" <- w2
  "?" <- w2
  "?" <- w2
  "?" <- w1
  "?" <- w1
  "?" <- w1
  "?" <- w1
  "?" <- w1
  "?" <- w1
  "?" <- w1
  "?" <- w1
  "?" <- w1
  "?" <- w1
  "?" <- w1
  "?" <- w1
  "?" <- w1
  "?" <- w1
  "?" <- w2
  "?" <- w2
  "?" <- w2
  "?" <- w2
  "?" <- w2
  "?" <- w2
  "?" <- w2
  "?" <- w2
  "?" <- w2
  "?" <- w2
  "?" <- w2
  "?" <- w2
  "?" <- w2
  "?" <- w2
  "?" <- w2
  "?" <- w2
  "?" <- w2
  "?" <- w2
  "?" <- w1
  "?" <- w1
  "?" <- w1
  "?" <- w1
  "?" <- w1
  "?" <- w1
  "?" <- w1
  "?" <- w1
  "?" <- w1
  "?" <- w1
  "?" <- w1
  "?" <- w1
  "?" <- w1
  "?" <- w1
  "?" <- w1
  "?" <- w1
  "?" <- w1
  "?" <- w1
  "?" <- w1
  "?" <- w1
  "?" <- w1
  "?" <- w1
  "?" <- w1
